vi "StreamTransmitSyncBox.vi"() -> ()   [LabVIEW 2018]
panel:
  out "error out":errorcluster
  in  "stop":bool
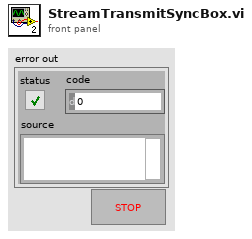
[diagram p1: front panel]
types:
  T1 = cluster{"ID":u32, "Address":string, "Service Name 1":string, "Service Name 2":string, "queue TX":refnum<queue>, "queue RX":refnum<queue>, "Port 1":u32, "Port 2":u32}
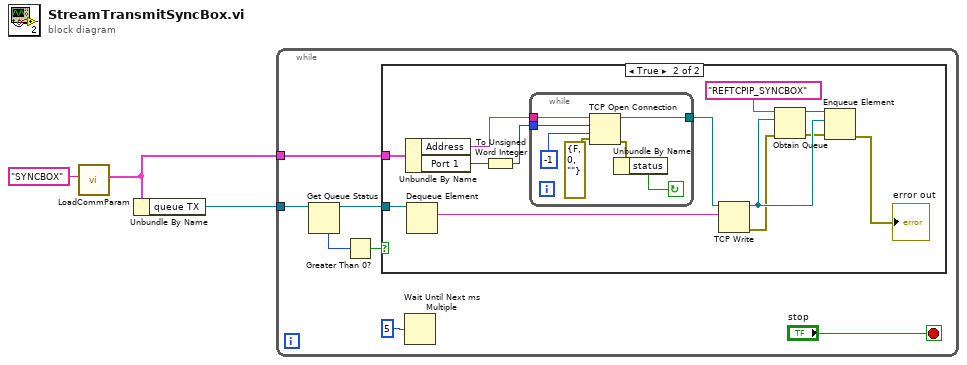
[diagram p0: block diagram]
diagram:
  n1 = call "LoadCommParam.vi"("section name"="SYNCBOX") -> ("output cluster"=w1:T1)  [unwired: 10 in]
  n2 = Unbundle By Name(w1) -> ("queue TX"=w2:refnum<queue>)
  n3 = while {
    tunnel: w2 -> [w10]
    tunnel: w1 -> [w5]
    stop <- "stop" stop-if-true
    n4 = Get Queue Status(queue=w10) -> (queue out=w7:refnum<queue>, # elements in queue=w9:i32)  [unwired: 2 in, 6 out]
    n5 = Greater Than 0?(x=w9) -> (x > 0?=w8:bool)
    n6 = case shown="True" w8 {
      tunnel: w7 -> [_ w23]
      tunnel: w5 -> [_ w21]
      frame False {
      }
      frame True {
        n7 = Unbundle By Name(w21) -> ("Address"=w20:string, "Port 1"=w19:u32)
        n8 = Dequeue Element(queue=w23) -> (element=w22:string)  [unwired: 2 in, 3 out]
        n9 = To Unsigned Word Integer(number=w19) -> (unsigned 16bit integer=w18:u16)
        n10 = while {
          tunnel: w20 -> [w30]
          tunnel: w18 -> [w29]
          tunnel: [w28] -> w17
          stop <- w25 continue-if-true
          n11 = TCP Open Connection(address=w30, remote port or service name=w29, timeout ms (60000)=-1, error in (no error)=errorcluster {"status"=FALSE, "code"=0, "source"=""}) -> (connection ID=w28:refnum<k5>, error out=w26:errorcluster)  [unwired: 1 in]
          n12 = Unbundle By Name(w26) -> ("status"=w25:bool)
        }
        n13 = TCP Write(connection ID=w17, data in=w22) -> (connection ID out=w14:refnum<k5>, error out=w13:errorcluster)  [unwired: 2 in, 1 out]
        n14 = Obtain Queue(name (unnamed)="REFTCPIP_SYNCBOX", element data type=w14, error in (no error)=w13) -> (queue out=w16:refnum<queue>, error out=w12:errorcluster)  [unwired: 2 in, 1 out]
        n15 = Enqueue Element(queue=w16, element=w14, error in (no error)=w12) -> (error out=→"error out":errorcluster)  [unwired: 1 in, 2 out]
      }
    }
    n16 = Wait Until Next ms Multiple(millisecond multiple=u32 5) -> ()  [unwired: 1 out]
  }
